vi "test_parseRangeMode.vi"(8 "error in (no error)":errorcluster) -> (0 "error out":errorcluster)   [LabVIEW 2020, in "horiba.test.lvlib"]
uses:
  horiba.test.lvlib
  <vilib>/addons/_JKI Toolkits/Caraya/classes/Test/Test.lvclass
  <vilib>/addons/_JKI Toolkits/Caraya/classes/Assert/Assert.lvclass
  Classes/CCD/CCD.lvclass
  <vilib>/addons/_JKI Toolkits/Caraya/classes/Assert/Assert Not Error.vi
  <vilib>/addons/_JKI Toolkits/Caraya/classes/Assert/Assert Equal Value and Type_Variant.vi
panel:
  # "Connector Pane"
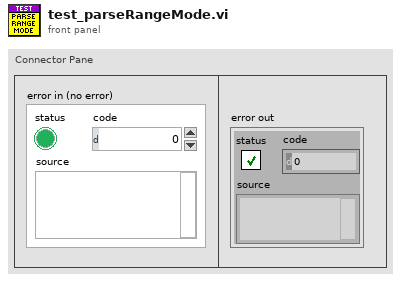
[diagram p1: front panel]
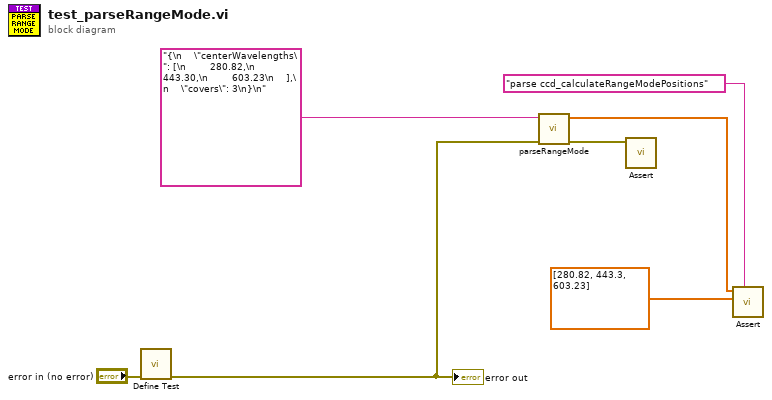
[diagram p0: block diagram]
diagram:
  n1 = call <vilib>:"Define Test.vi"("error in (no error)"="error in (no error)") -> ("error out"=w2:errorcluster)  [unwired: 9 in, 1 out]
  "error out" <- w2
  n2 = call "parseRangeMode.vi"("error in (no error)"=w2, "String"="{\n    \"centerWavelengths\": [\n        280.82,\n        443.30,\n        603.23\n    ],\n    \"covers\": 3\n}\n") -> ("error out"=w1:errorcluster, "Data"=w4:dbl[])  [unwired: 8 in]
  n3 = call-poly <vilib>:"Assert.vi"("Not Error?"=w1) -> ()  [unwired: 9 in, 2 out]
  n4 = call-poly <vilib>:"Assert.vi"("Label"="parse ccd_calculateRangeModePositions" ("Label (VI Title)"), "Y"=dbl[] [280.82, 443.3, 603.23], "X"=w4) -> ()  [unwired: 7 in, 2 out]
